vi "sc_relXYZ_steps.vi"(0 "VISA handle":refnum<visa-resource-name>, 5 "rel X dist (steps)":i32, 7 "rel Y dist (steps)":i32, 9 "rel Z dist (steps)":i32, 11 "error in (no error)":errorcluster) -> (4 "Dup. VISA handle":refnum<visa-resource-name>, 15 "error out":errorcluster)   [LabVIEW 2015]
uses:
  controls/scientifica_commands.ctl
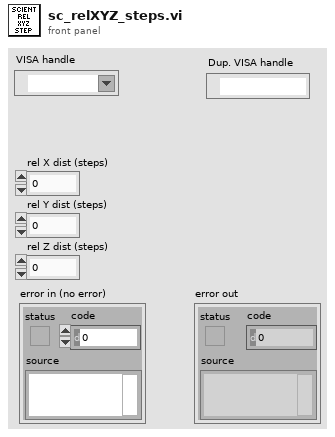
[diagram p1: front panel]
types:
  T1 = typedef "scientifica_commands.ctl" = enum16{"ANGLE", "INSET", "FIRST", "ZERO", "Pz", "P", "absz", "ACC", "TOP", "STOP", "rel", "relz", "abs", "IN", "vj", "APROACH", "OBJS", "OBJU", "OUT", "OBJ", "OBJL", "SET", "OBJD", "STEP", "SETSTEP", "S", "UUX", "UUY", "UUZ"}
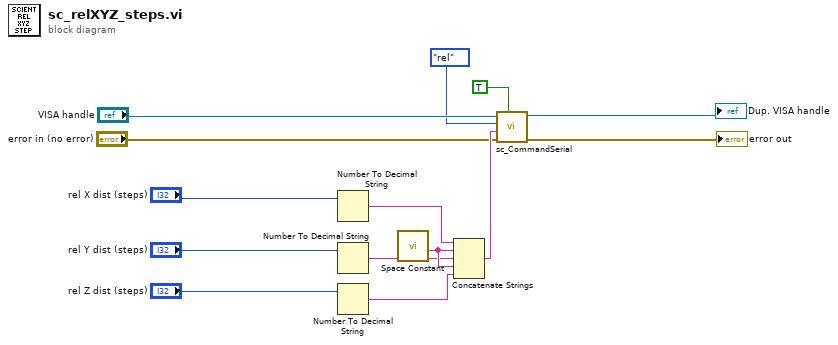
[diagram p0: block diagram]
diagram:
  n1 = Number To Decimal String(number="rel X dist (steps)") -> (decimal integer string=w7:string)  [unwired: 1 in]
  n2 = Number To Decimal String(number="rel Y dist (steps)") -> (decimal integer string=w8:string)  [unwired: 1 in]
  n3 = Number To Decimal String(number="rel Z dist (steps)") -> (decimal integer string=w13:string)  [unwired: 1 in]
  n4 = call <vilib>:"Space Constant.vi"() -> ("String"=w12:string)
  n5 = Concatenate Strings(w7, w12, w8, w12, w13) -> (w14:string)
  n6 = call "sc_CommandSerial.vi"("Query?"=TRUE, "error in (no error)"="error in (no error)", "argument"=w14, "Scientifica commands"=scientifica_commands."rel", "VISA handle"="VISA handle") -> ("error out"=→"error out":errorcluster, "Dup. VISA handle"=→"Dup. VISA handle":refnum<visa-resource-name>)  [unwired: 3 in, 2 out]
